vi "op.vi"(8 "initialized array":dbl[](array[numeric]), 9 "delay":i32, 11 "Xwe":dbl) -> (0 "s? t:f":dbl[](array[numeric]), 3 "Xwy":dbl)   [LabVIEW 2019]
panel:
  out "Waveform Chart":cluster{"X0":dbl, "Xwe":dbl}(graph)
  out "Larger that delay":bool
  out "Equal to delay":bool
  out "delay res":i32
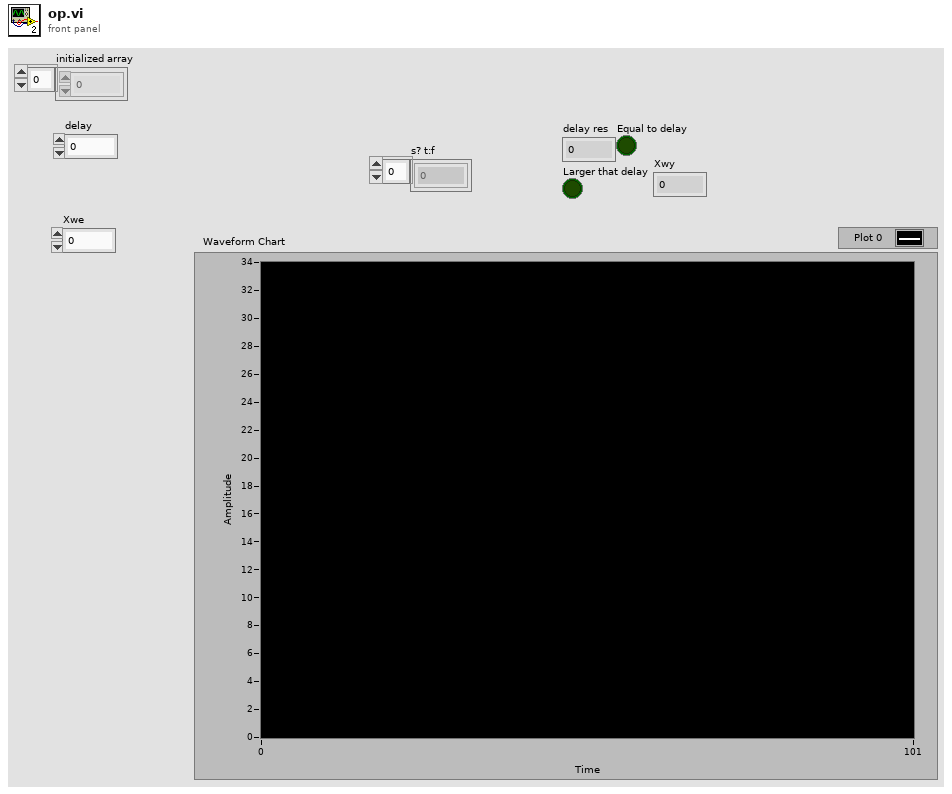
[diagram p1: front panel]
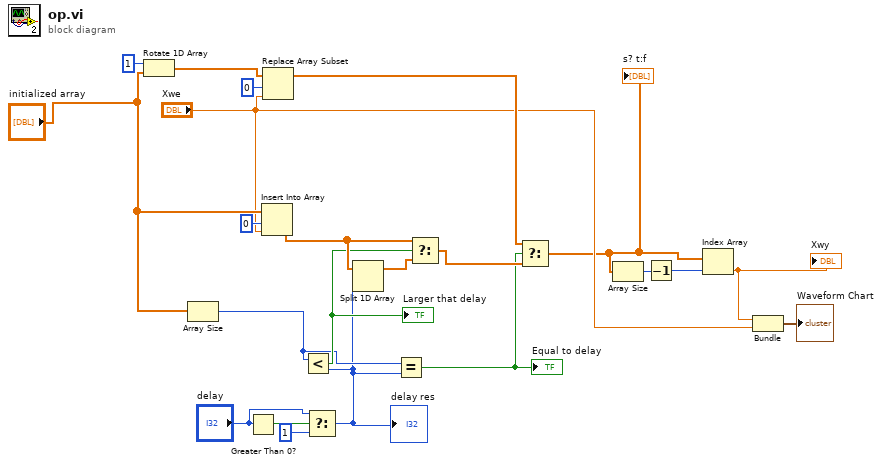
[diagram p0: block diagram]
diagram:
  n1 = Rotate 1D Array(1:"initialized array", 2:1 ("n")) -> (0:w21:dbl[])
  n2 = Array Size(array="initialized array") -> (size(s)=w12:i32)
  n3 = Greater Than 0?(x="delay") -> (x > 0?=w15:bool)
  n4 = Insert Into Array(array="initialized array", index=0, new element="Xwe") -> (w17:dbl[])
  n5 = Replace Array Subset(array=w21, new element="Xwe", index=0) -> (w9:dbl[])
  n6 = Select(t="delay", s=w15, f=1) -> (s? t:f=w11:i32)
  "delay res" <- w11
  n7 = Less?(x=w12, y=w11) -> (x < y?=w13:bool)
  "Larger that delay" <- w13
  n8 = Split 1D Array(array=w17, index=w11) -> (first subarray=w16:dbl[])  [unwired: 1 out]
  n9 = Equal?(x=w12, y=w11) -> (x = y?=w8:bool)
  "Equal to delay" <- w8
  n10 = Select(t=w17, s=w13, f=w16) -> (s? t:f=w10:dbl[])
  n11 = Select(t=w9, s=w8, f=w10) -> (s? t:f=w1:dbl[])
  "s? t:f" <- w1
  n12 = Array Size(array=w1) -> (size(s)=w7:i32)
  n13 = Decrement(x=w7) -> (x-1=w6:i32)
  n14 = Index Array(array=w1, index=w6) -> (element=w5:dbl)
  "Xwy" <- w5
  n15 = Bundle("X0"=w5, "Xwe"="Xwe") -> (→"Waveform Chart":cluster{"X0":dbl, "Xwe":dbl})  [unwired: 1 in]
